vi "PH_Tektronix_7000.Evt Call Set Channel Name.vi"(0 "i ref in":refnum<vi>, 1 "Instance":string="N/A", 2 "Channel":u16(ring) items=["Channel 1", "Channel 2", "Channel 3", "Channel 4", "Math 1", "Math 2", "Math 3", "Math 4", "Reference 1", "Reference 2", "Reference 3", "Reference 4"], 3 "Channel Name":string="N/A", 5 "error in (no error)":errorcluster) -> (14 "i ref out":refnum<vi>, 19 "error out":errorcluster)   [LabVIEW 2014, in "PH_Tektronix_7000.lvlib"]
doc: "This VI calls sets a simple call."
uses:
  PH_Tektronix_7000.lvlib
  CS_Core/CSSystem/CoreLib/CoreLib.string 2 byte array.vi
  CS_Core/CSSystem/CoreLib/CoreLib.short 2 byte array.vi
  CS_Core/CSSystem/CoreLib/CoreLib.lvlib
  CS_Core/BaseProcess/BaseProcess.lvlib
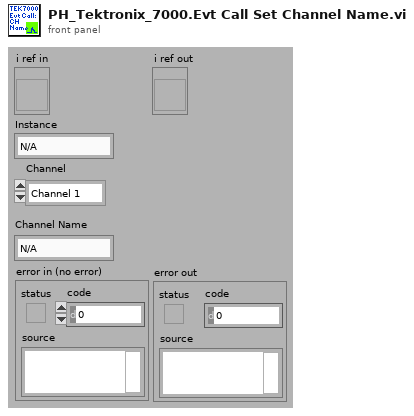
[diagram p1: front panel]
types:
  T1 = typedef "CoreDefs.rawDataType.ctl" = i8[]
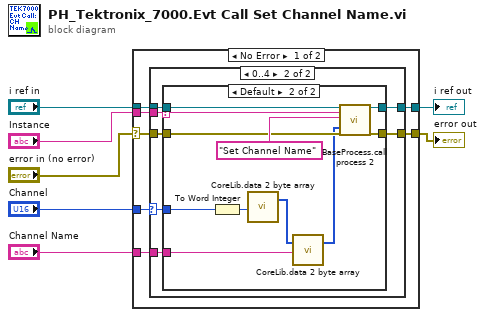
[diagram p0: block diagram]
diagram:
  n1 = case shown="No Error" "error in (no error)" {
    selector: "error in (no error)" -> [w10 w37]
    tunnel: [w14 w38] -> w7
    tunnel: [w13 w37] -> w6
    tunnel: "i ref in" -> [w12 w38]
    tunnel: "Channel" -> [w9 _]
    tunnel: "Instance" -> [w11 _]
    tunnel: "Channel Name" -> [w8 _]
    frame No Error {
      n2 = case shown="0..4" w9 {
        selector: w9 -> [_ w18]
        tunnel: [w16 w23] -> w14
        tunnel: [w15 w22] -> w13
        tunnel: w12 -> [w16 w21]
        tunnel: w11 -> [_ w20]
        tunnel: w10 -> [w15 w19]
        tunnel: w8 -> [_ w17]
        frame Default {
        }
        frame 0..4 {
          n3 = case shown="Default" w20 {
            selector: w20 -> [_ w31]
            tunnel: [w24 w35] -> w23
            tunnel: [w25 w34] -> w22
            tunnel: w21 -> [w24 w33]
            tunnel: w19 -> [w25 w32]
            tunnel: w18 -> [_ w30]
            tunnel: w17 -> [_ w26]
            frame "N/A" {
            }
            frame Default {
              n4 = To Word Integer(number=w30) -> (16bit integer=w28:i16)
              n5 = call-poly "CoreLib.data 2 byte array.vi"("i16"=w28) -> ("byteArray out"=w29:T1)  [unwired: 18 in]
              n6 = call-poly "CoreLib.data 2 byte array.vi"("byteArray"=w29, "string"=w26) -> ("byteArray out"=w27:T1)  [unwired: 17 in]
              n7 = call "BaseProcess.call process 2.vi"("i ref in"=w33, "Object"=w31, "Selector"="Set Channel Name", "Data"=w27, "error in (no error)"=w32) -> ("i ref out"=w35:refnum<vi>, "error out"=w34:errorcluster)  [unwired: 13 in]
            }
          }
        }
      }
    }
    frame Error {
    }
  }
  "i ref out" <- w7
  "error out" <- w6
